vi "Excercise 3-6.vi"() -> ()   [LabVIEW 2014]
panel:
  out "Converted Temperature":dbl
  in  "Original Temperature":dbl
  in  "STOP":bool
  in  "Mode":T1(ring)
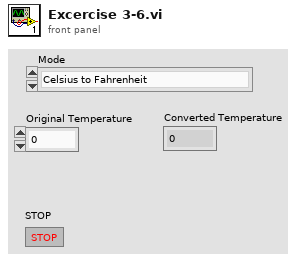
[diagram p1: front panel]
types:
  T1 = enum16{"Celsius to Fahrenheit", "Fahrenheit to Celsius", "Celsius to Kelvin", "Fahrenheit to Kelvin"}
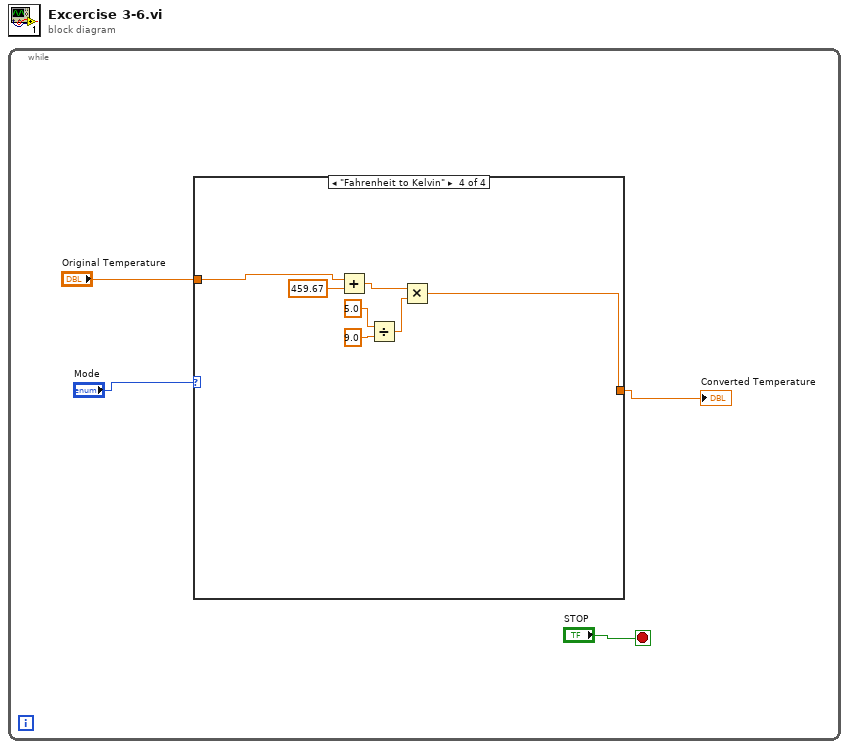
[diagram p0: block diagram]
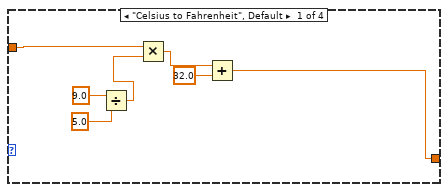
[diagram p2: hidden frame]
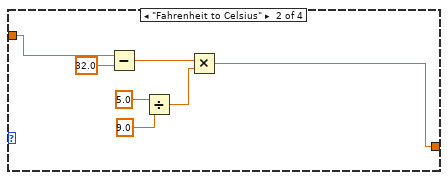
[diagram p3: hidden frame]
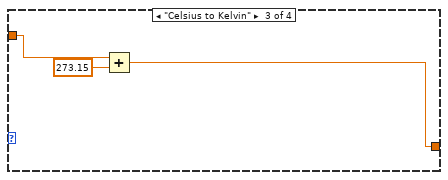
[diagram p4: hidden frame]
diagram:
  n1 = while {
    stop <- "STOP" stop-if-true
    n2 = case shown="\"Fahrenheit to Kelvin\"" "Mode" {
      tunnel: [w5 w12 w19 w23] -> w2
      tunnel: "Original Temperature" -> [w11 w18 w21 w22]
      frame "Celsius to Fahrenheit", Default {
        n3 = Divide(x=9.0, y=5.0) -> (x/y=w10:dbl)
        n4 = Multiply(x=w11, y=w10) -> (x*y=w7:dbl)
        n5 = Add(x=w7, y=32.0) -> (x+y=w5:dbl)
      }
      frame "Fahrenheit to Celsius" {
        n6 = Subtract(x=w18, y=32.0) -> (x-y=w16:dbl)
        n7 = Divide(x=5.0, y=9.0) -> (x/y=w15:dbl)
        n8 = Multiply(x=w16, y=w15) -> (x*y=w12:dbl)
      }
      frame "Celsius to Kelvin" {
        n9 = Add(x=w21, y=273.15) -> (x+y=w19:dbl)
      }
      frame "Fahrenheit to Kelvin" {
        n10 = Add(x=w22, y=459.67) -> (x+y=w27:dbl)
        n11 = Divide(x=5.0, y=9.0) -> (x/y=w26:dbl)
        n12 = Multiply(x=w27, y=w26) -> (x*y=w23:dbl)
      }
    }
    "Converted Temperature" <- w2
  }
